vi "Move_2_tl.vi"(3 "Target Position":i32 step=1) -> (0 "Move OK?":bool, 1 "Current Position":i32)   [LabVIEW 2010]
uses:
  Traverse_setup_tl.glob.vi
panel:
  in  "Case Constant\n(See Context Help)":bool
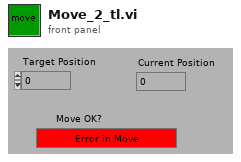
[diagram p1: front panel]
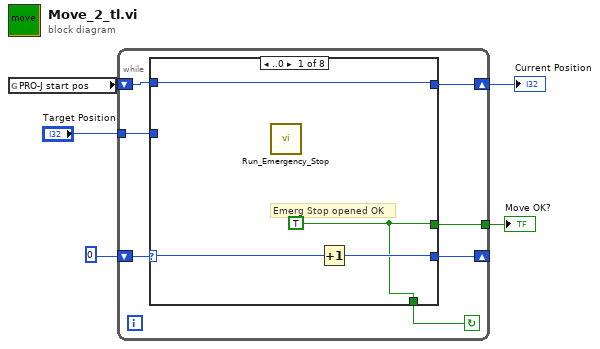
[diagram p0: block diagram]
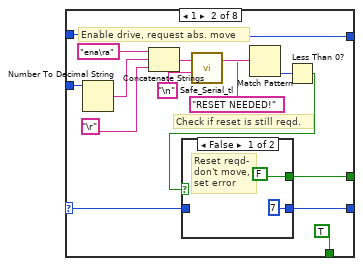
[diagram p2: hidden frame]
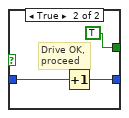
[diagram p3: hidden frame]
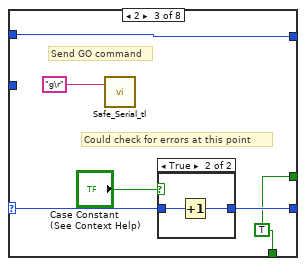
[diagram p4: hidden frame]
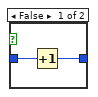
[diagram p5: hidden frame]
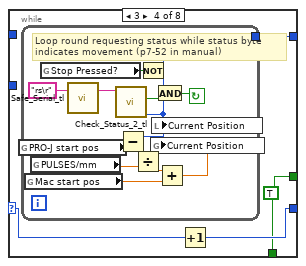
[diagram p6: hidden frame]
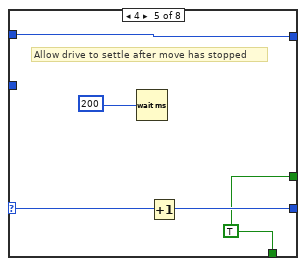
[diagram p7: hidden frame]
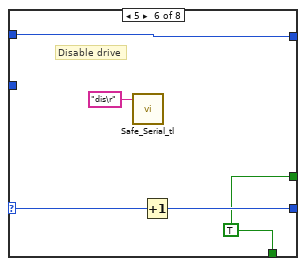
[diagram p8: hidden frame]
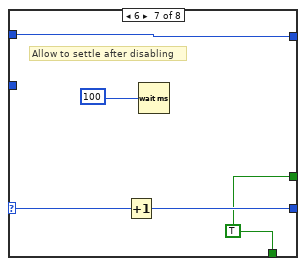
[diagram p9: hidden frame]
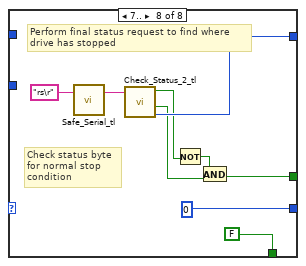
[diagram p10: hidden frame]
diagram:
  n1 = global read "Traverse_setup_tl.glob.vi" "PRO-J start pos"() -> (w1:i32)
  n2 = while {
    tunnel: [w7] -> w2
    shift-left: w1 -> [w9]
    shift-right: [w6] -> w3
    shift-left: 0 -> [w11]
    shift-right: [w10] -> _
    tunnel: "Target Position" -> [w12]
    stop <- w8 continue-if-true
    n3 = case shown="..0" w11 {
      tunnel: w12 -> [_ w29 _ _ _ _ _ _]
      tunnel: [w16 w21 w38 w48 w65 w70 w75 w83] -> w6
      selector: w11 -> [w15 w23 w42 w47 w67 w72 w77 _]
      tunnel: [w14 w22 w41 w50 w66 w71 w76 0] -> w10
      tunnel: w9 -> [w16 w21 w38 _ w65 w70 w75 _]
      tunnel: [w13 TRUE w37 w49 w64 w69 w74 FALSE] -> w8
      tunnel: [w13 w19 w37 w49 w64 w69 w74 w79] -> w7
      frame ..0 {
        w13 = TRUE
        # "Emerg Stop opened OK"
        n4 = call "Run_Emergency_Stop.vi"() -> ()  [unwired: 8 in]
        n5 = Increment(x=w15) -> (x+1=w14:i32)
      }
      frame 1 {
        # "Check if reset is still reqd."
        # "Enable drive, request abs. move"
        n6 = Number To Decimal String(number=w29) -> (decimal integer string=w30:string)  [unwired: 1 in]
        n7 = Concatenate Strings("ena\ra", w30, "\r") -> (w28:string)
        n8 = call "Safe_Serial_tl.vi"("Tx String"=w28, "Terminator (glob)"="\n") -> ("Rx String"=w25:string)  [unwired: 4 in, 1 out]
        n9 = Match Pattern(string=w25, regular expression="RESET NEEDED!") -> (offset past match=w27:i32)  [unwired: 1 in, 3 out]
        n10 = Less Than 0?(x=w27) -> (x < 0?=w24:bool)
        n11 = case shown="False" w24 {
          tunnel: w23 -> [_ w36]
          tunnel: [7 w35] -> w22
          tunnel: [FALSE TRUE] -> w19
          frame False {
            # "Reset reqd-\ndon't move,\nset error"
          }
          frame True {
            # "Drive OK,\nproceed"
            n12 = Increment(x=w36) -> (x+1=w35:i32)
          }
        }
      }
      frame 2 {
        w37 = TRUE
        # "Could check for errors at this point"
        # "Send GO command"
        n13 = call "Safe_Serial_tl.vi"("Tx String"="g\r") -> ()  [unwired: 5 in, 2 out]
        n14 = case shown="True" "Case Constant\n(See Context Help)" {
          tunnel: w42 -> [w44 w46]
          tunnel: [w43 w45] -> w41
          frame False {
            n15 = Increment(x=w44) -> (x+1=w43:i32)
          }
          frame True {
            n16 = Increment(x=w46) -> (x+1=w45:i32)
          }
        }
      }
      frame 3 {
        w49 = TRUE
        n17 = while {
          tunnel: [w55] -> w48
          stop <- w51 continue-if-true
          # "Loop round requesting status while status byte\nindicates movement (p7-52 in manual)"
          n18 = global read "Traverse_setup_tl.glob.vi" "PRO-J start pos"() -> (w61:i32)
          n19 = global read "Traverse_setup_tl.glob.vi" "Mac start pos"() -> (w58:dbl)
          n20 = global read "Traverse_setup_tl.glob.vi" "PULSES/mm"() -> (w59:dbl)
          n21 = global read "Traverse_setup_tl.glob.vi" "Stop Pressed?"() -> (w54:bool)
          n22 = call "Safe_Serial_tl.vi"("Tx String"="rs\r") -> ("Rx String"=w62:string)  [unwired: 5 in, 1 out]
          n23 = call "Check_Status_2_tl.vi"("Status Request Reply"=w62) -> ("Keep Checking?"=w52:bool, "Current Position"=w55:i32)  [unwired: 3 out]
          n24 = Subtract(x=w55, y=w61) -> (x-y=w60:i32)
          n25 = Divide(x=w60, y=w59) -> (x/y=w57:dbl)
          n26 = Not(x=w54) -> (.not. x?=w53:bool)
          n27 = local write "Current Position"(w55) -> ()
          n28 = And(x=w53, y=w52) -> (x .and. y?=w51:bool)
          n29 = Add(x=w57, y=w58) -> (x+y=w56:dbl)
          n30 = global write "Traverse_setup_tl.glob.vi" "Current Position"(w56) -> ()
        }
        n31 = Increment(x=w47) -> (x+1=w50:i32)
      }
      frame 4 {
        w64 = TRUE
        # "Allow drive to settle after move has stopped"
        n32 = Wait (ms)(milliseconds to wait=200) -> ()  [unwired: 1 out]
        n33 = Increment(x=w67) -> (x+1=w66:i32)
      }
      frame 5 {
        w69 = TRUE
        # "Disable drive"
        n34 = call "Safe_Serial_tl.vi"("Tx String"="dis\r") -> ()  [unwired: 5 in, 2 out]
        n35 = Increment(x=w72) -> (x+1=w71:i32)
      }
      frame 6 {
        w74 = TRUE
        # "Allow to settle after disabling"
        n36 = Increment(x=w77) -> (x+1=w76:i32)
        n37 = Wait (ms)(milliseconds to wait=100) -> ()  [unwired: 1 out]
      }
      frame 7.. {
        # "Check status byte\nfor normal stop\ncondition"
        # "Perform final status request to find where\ndrive has stopped"
        n38 = call "Safe_Serial_tl.vi"("Tx String"="rs\r") -> ("Rx String"=w84:string)  [unwired: 5 in, 1 out]
        n39 = call "Check_Status_2_tl.vi"("Status Request Reply"=w84) -> ("Error?"=w81:bool, "Stopped?"=w82:bool, "Current Position"=w83:i32)  [unwired: 2 out]
        n40 = Not(x=w81) -> (.not. x?=w80:bool)
        n41 = And(x=w80, y=w82) -> (x .and. y?=w79:bool)
      }
    }
  }
  "Current Position" <- w3
  "Move OK?" <- w2
